vi "solar_misc Netstat.vi"() -> ()   [LabVIEW 2018]
doc: "This user interface displays TCP port statuses using the 'netstat' command line prompt. This is useful to ensure the ports are closed properly and if TCP ports have a 'CLOSE_WAIT' that rejects a new TCP connection."
panel:
  out "Update":dbl format="%.3f sec"
  in  "Filter State":string
  in  "Filter Port":string
  in  "Filter IP":string
  in  "Update Rate":dbl=1.0 format="%#.3f sec"
  in  "MCLB":i32(listbox)
  out "error out":errorcluster
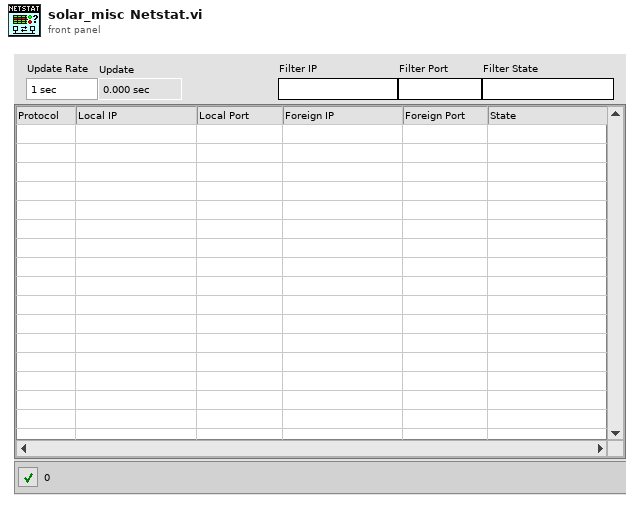
[diagram p1: front panel]
types:
  T1 = cluster{"Protocol":enum16{"invalid", "tcp", "udp", "icmp", "ip", "tcpv6", "udpv6", "icmpv6", "ipv6"}, "LocalIP":string, "LocalPort":u16, "ForeignIP":string, "ForeignPort":u16, "State":enum8{"UNKNOWN", "LISTEN", "ESTABLISHED", "SYN_SENT", "SYN_RECV", "LAST_ACK", "CLOSE_WAIT", "TIME_WAIT", "CLOSED", "CLOSING", "FIN_WAIT1", "FIN_WAIT2"}}[]
  T2 = enum8{"UNKNOWN", "LISTEN", "ESTABLISHED", "SYN_SENT", "SYN_RECV", "LAST_ACK", "CLOSE_WAIT", "TIME_WAIT", "CLOSED", "CLOSING", "FIN_WAIT1", "FIN_WAIT2"}
  T3 = enum16{"invalid", "tcp", "udp", "icmp", "ip", "tcpv6", "udpv6", "icmpv6", "ipv6"}
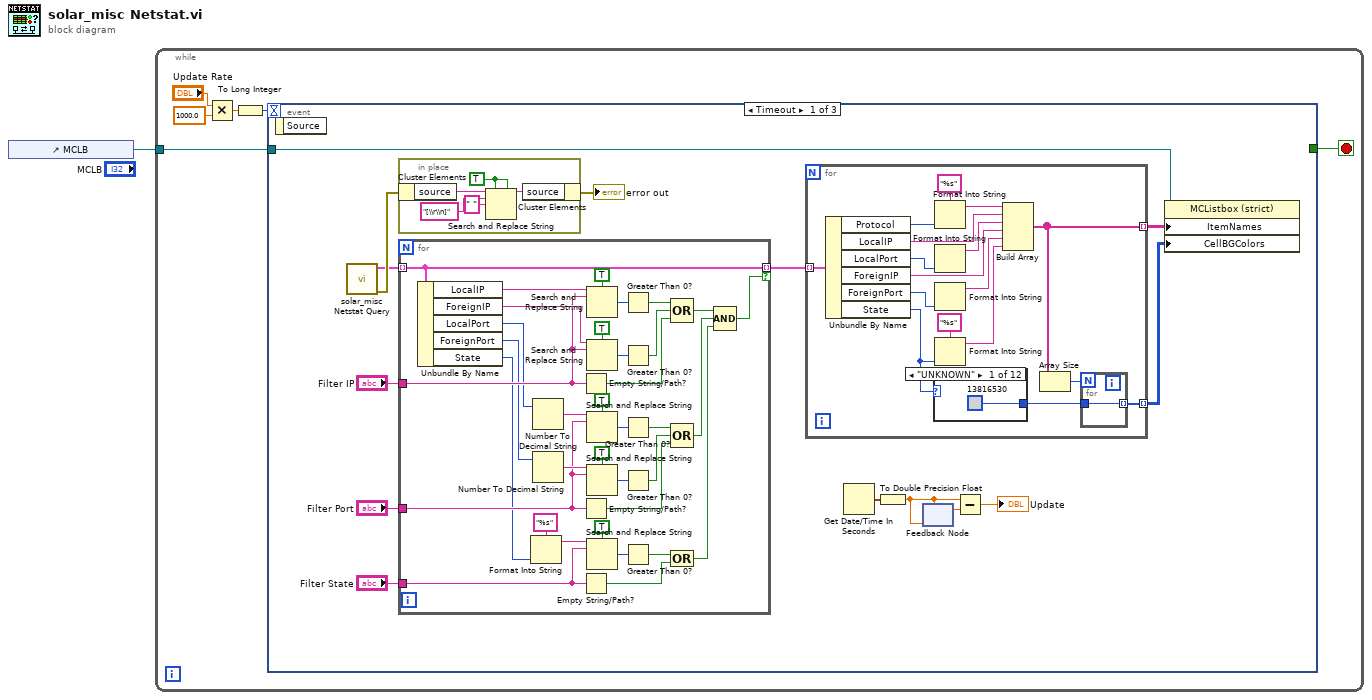
[diagram p0: block diagram]
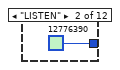
[diagram p2: hidden frame]
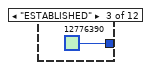
[diagram p3: hidden frame]
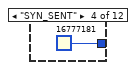
[diagram p4: hidden frame]
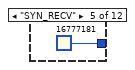
[diagram p5: hidden frame]
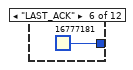
[diagram p6: hidden frame]
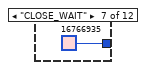
[diagram p7: hidden frame]
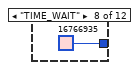
[diagram p8: hidden frame]
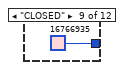
[diagram p9: hidden frame]
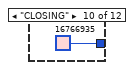
[diagram p10: hidden frame]
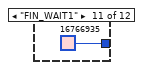
[diagram p11: hidden frame]
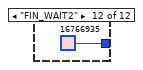
[diagram p12: hidden frame]
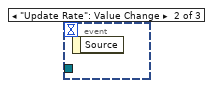
[diagram p13: hidden frame]
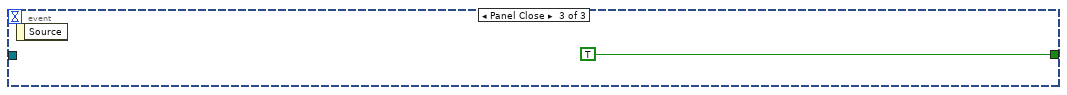
[diagram p14: hidden frame]
diagram:
  n1 = control-ref of="MCLB"() -> (w1:refnum<vi>)
  n2 = while {
    tunnel: w1 -> [w3]
    stop <- w2 stop-if-true
    n3 = Multiply(x="Update Rate", y=1000.0 ("x")) -> (x*y=w5:dbl)
    n4 = To Long Integer(number=w5) -> (32bit integer=w4:i32)
    n5 = event shown="[0] Timeout" {
      selector: _ -> [_ _ _]
      dyn-events: _ -> [_ _ _]
      timeout: w4 -> [_ _ _]
      tunnel: w3 -> [w18 _ _]
      tunnel: [_ _ TRUE] -> w2
      event Timeout {
        n6 = event-data() -> ()  [unwired: 1 in, 1 out]
        n7 = call "solar_misc Netstat Query.vi"() -> ("error out"=w20:errorcluster, "netstat"=w16:T1)  [unwired: 10 in]
        n8 = in-place {
          w87 = TRUE ("replace all? (F)")
          n9 = in-place-cluster #1(w20) -> ("source"=w91:string)
          n10 = Search and Replace String(replace all?=w87, multiline?=w87, input string=w91, search string="[\\r\\n]", replace string=" " ("replace string (\"\")")) -> (result string=w90:string)  [unwired: 3 in, 3 out]
          n11 = in-place-cluster #1("source"=w90) -> (→"error out":errorcluster)
        }
        n12 = for {
          tunnel: w16 -> [w45] mode=indexing
          tunnel: "Filter IP" -> [w48]
          tunnel: [w45] -> w15 mode=indexing if=w44
          tunnel: "Filter Port" -> [w32]
          tunnel: "Filter State" -> [w24]
          n13 = Unbundle By Name(w45) -> ("LocalIP"=w54:string, "ForeignIP"=w53:string, "LocalPort"=w36:u16, "ForeignPort"=w34:u16, "State"=w27:T2)
          n14 = Format Into String(format string="%s", w27) -> (resulting string=w25:string)  [unwired: 2 in, 1 out]
          n15 = Number To Decimal String(number=w36) -> (decimal integer string=w35:string)  [unwired: 1 in]
          n16 = Number To Decimal String(number=w34) -> (decimal integer string=w33:string)  [unwired: 1 in]
          n17 = Empty String/Path?(string/path=w48) -> (empty?=w47:bool)
          n18 = Empty String/Path?(string/path=w32) -> (empty?=w43:bool)
          n19 = Empty String/Path?(string/path=w24) -> (empty?=w28:bool)
          n20 = Search and Replace String(case sensitive?=TRUE ("ignore case? (F)"), input string=w54, search string=w48) -> (number of replacements=w52:i32)  [unwired: 5 in, 3 out]
          n21 = Search and Replace String(case sensitive?=TRUE ("ignore case? (F)"), input string=w53, search string=w48) -> (number of replacements=w51:i32)  [unwired: 5 in, 3 out]
          n22 = Search and Replace String(case sensitive?=TRUE ("ignore case? (F)"), input string=w35, search string=w32) -> (number of replacements=w39:i32)  [unwired: 5 in, 3 out]
          n23 = Search and Replace String(case sensitive?=TRUE ("ignore case? (F)"), input string=w33, search string=w32) -> (number of replacements=w40:i32)  [unwired: 5 in, 3 out]
          n24 = Search and Replace String(case sensitive?=TRUE ("ignore case? (F)"), input string=w25, search string=w24) -> (number of replacements=w30:i32)  [unwired: 5 in, 3 out]
          n25 = Greater Than 0?(x=w52) -> (x > 0?=w50:bool)
          n26 = Greater Than 0?(x=w51) -> (x > 0?=w49:bool)
          n27 = Greater Than 0?(x=w39) -> (x > 0?=w41:bool)
          n28 = Greater Than 0?(x=w40) -> (x > 0?=w42:bool)
          n29 = Greater Than 0?(x=w30) -> (x > 0?=w29:bool)
          n30 = Compound Arithmetic op=OR(w50, w49, w47) -> (w46:bool)
          n31 = Compound Arithmetic op=OR(w41, w42, w43) -> (w23:bool)
          n32 = Compound Arithmetic op=OR(w29, w28) -> (w22:bool)
          n33 = Compound Arithmetic op=AND(w46, w23, w22) -> (w44:bool)
        }
        n34 = for {
          tunnel: w15 -> [w73] mode=indexing
          tunnel: [w59] -> w19 mode=indexing
          tunnel: [w57] -> w17 mode=indexing
          n35 = Unbundle By Name(w73) -> ("Protocol"=w72:T3, "LocalIP"=w69:string, "LocalPort"=w68:u16, "ForeignIP"=w66:string, "ForeignPort"=w65:u16, "State"=w61:T2)
          n36 = case shown="\"UNKNOWN\"" w61 {
            tunnel: [u32 13816530 u32 12776390 u32 12776390 u32 16777181 u32 16777181 u32 16777181 u32 16766935 u32 16766935 u32 16766935 u32 16766935 u32 16766935 u32 16766935] -> w60
            frame "UNKNOWN" {
            }
            frame "LISTEN" {
            }
            frame "ESTABLISHED" {
            }
            frame "SYN_SENT" {
            }
            frame "SYN_RECV" {
            }
            frame "LAST_ACK" {
            }
            frame "CLOSE_WAIT" {
            }
            frame "TIME_WAIT" {
            }
            frame "CLOSED" {
            }
            frame "CLOSING" {
            }
            frame "FIN_WAIT1" {
            }
            frame "FIN_WAIT2" {
            }
          }
          n37 = Format Into String(format string="%s", w72) -> (resulting string=w70:string)  [unwired: 2 in, 1 out]
          n38 = Format Into String(w68) -> (resulting string=w67:string)  [unwired: 3 in, 1 out]
          n39 = Format Into String(w65) -> (resulting string=w64:string)  [unwired: 3 in, 1 out]
          n40 = Format Into String(format string="%s", w61) -> (resulting string=w62:string)  [unwired: 2 in, 1 out]
          n41 = Build Array(w70, w69, w67, w66, w64, w62) -> (w59:string[])
          n42 = Array Size(array=w59) -> (size(s)=w58:i32)
          n43 = for {
            N: w58 -> [_]
            tunnel: w60 -> [w74]
            tunnel: [w74] -> w57 mode=indexing
          }
        }
        n44 = Get Date/Time In Seconds() -> (seconds since 1Jan1904=w11:timestamp)
        n45 = To Double Precision Float(number=w11) -> (double precision float=w9:dbl)
        n46 = feedback-in #2(w9) -> ()
        n47 = feedback #2(w9) -> (w10:dbl)
        n48 = Subtract(x=w9, y=w10) -> (x-y=→"Update":dbl)
        n49 = property class="MCListbox (strict)"(reference=w18, "ItemNames"=w19, "CellBGColors"=w17) -> ()  [unwired: 1 in, 2 out]
      }
      event "Update Rate": Value Change {
        n50 = event-data() -> ()  [unwired: 1 in, 1 out]
      }
      event Panel Close {
        n51 = event-data() -> ()  [unwired: 1 in, 1 out]
      }
    }
  }
